vi "geographic index Maze Input.vi"(9 "Direction":T1, 11 "Maze (0: Empty, -1: Enemy. 1: Teammate":i32[][](array[numeric])) -> (2 "element":i32)   [LabVIEW 2014, in "JFD_Common.lvlib"]
uses:
  Type Defs/Direction Enum.ctl
  JFD_Common.lvlib
  Type Defs/SB Type Defs.lvlib
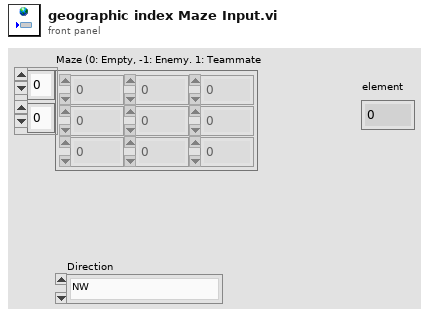
[diagram p1: front panel]
types:
  T1 = typedef "SB Type Defs.lvlib/Direction Enum.ctl" = enum16{"NW", "N", "NE", "E", "SE", "S", "SW", "W"}
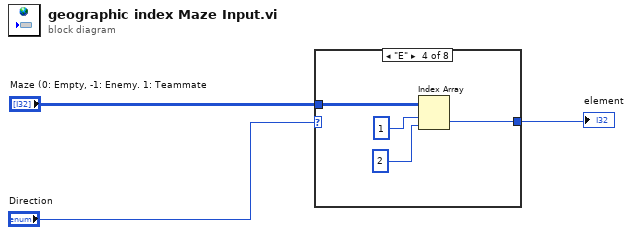
[diagram p0: block diagram]
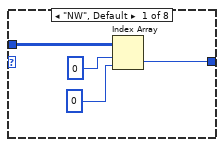
[diagram p2: hidden frame]
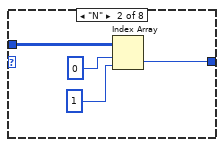
[diagram p3: hidden frame]
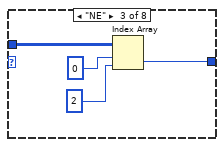
[diagram p4: hidden frame]
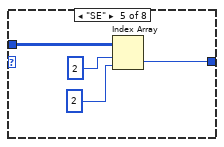
[diagram p5: hidden frame]
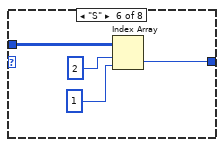
[diagram p6: hidden frame]
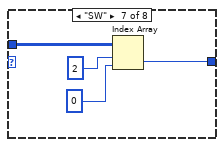
[diagram p7: hidden frame]
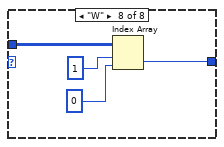
[diagram p8: hidden frame]
diagram:
  n1 = case shown="\"E\"" "Direction" {
    tunnel: "Maze (0: Empty, -1: Enemy. 1: Teammate" -> [w7 w11 w15 w19 w23 w27 w31 w35]
    tunnel: [w4 w8 w12 w16 w20 w24 w28 w32] -> w2
    frame "NW", Default {
      n2 = Index Array(array=w7, index (row)=0, index (col)=0 ("index (row)")) -> (element=w4:i32)
    }
    frame "N" {
      n3 = Index Array(array=w11, index (row)=0, index (col)=1 ("index (row)")) -> (element=w8:i32)
    }
    frame "NE" {
      n4 = Index Array(array=w15, index (row)=0, index (col)=2 ("index (row)")) -> (element=w12:i32)
    }
    frame "E" {
      n5 = Index Array(array=w19, index (row)=1, index (col)=2 ("index (row)")) -> (element=w16:i32)
    }
    frame "SE" {
      n6 = Index Array(array=w23, index (row)=2, index (col)=2 ("index (row)")) -> (element=w20:i32)
    }
    frame "S" {
      n7 = Index Array(array=w27, index (row)=2, index (col)=1 ("index (row)")) -> (element=w24:i32)
    }
    frame "SW" {
      n8 = Index Array(array=w31, index (row)=2, index (col)=0 ("index (row)")) -> (element=w28:i32)
    }
    frame "W" {
      n9 = Index Array(array=w35, index (row)=1, index (col)=0 ("index (row)")) -> (element=w32:i32)
    }
  }
  "element" <- w2
